vi "Abs.vi"(10 "Input":dbl[][](array[numeric]), 11 "Abs":bool) -> (2 "Array out":dbl[][](array[numeric]))   [LabVIEW 2018]
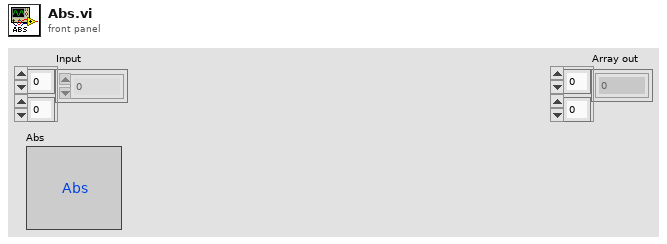
[diagram p1: front panel]
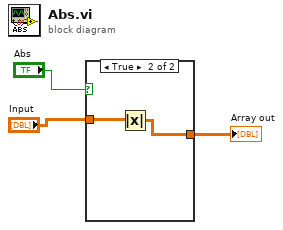
[diagram p0: block diagram]
diagram:
  n1 = case shown="True" "Abs" {
    tunnel: "Input" -> [w4 w6]
    tunnel: [w4 w5] -> w1
    frame False {
    }
    frame True {
      n2 = Absolute Value(x=w6) -> (abs(x)=w5:dbl[][])
    }
  }
  "Array out" <- w1
